vi "ADC_treat_data.vi"(1 "Inst_parameter":T1, 2 "data in":dbl[][](array[numeric])) -> (0 "data out":dbl[][](array[numeric]))   [LabVIEW 2013]
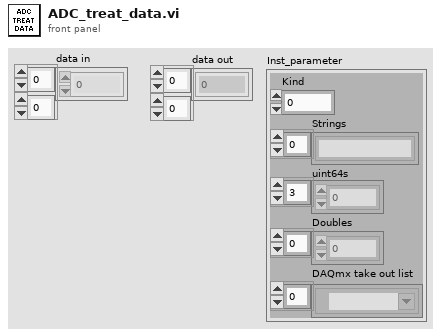
[diagram p1: front panel]
types:
  T1 = cluster{"Kind":u16, "Strings":string[], "uint64s":u64[], "Doubles":dbl[], "DAQmx take out list":refnum<k21>[]}
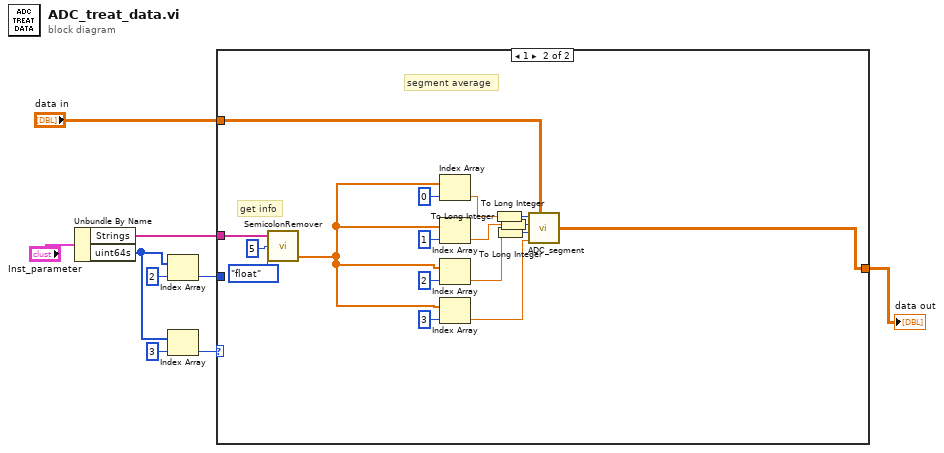
[diagram p0: block diagram]
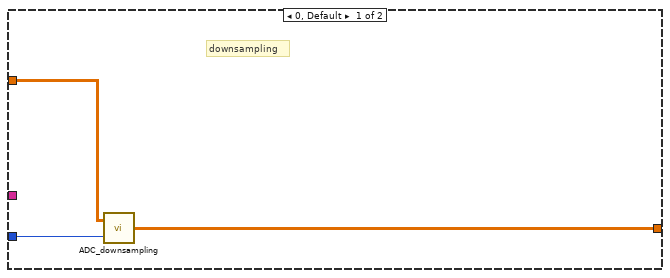
[diagram p2: hidden frame]
diagram:
  n1 = Unbundle By Name("Inst_parameter") -> ("Strings"=w6:string[], "uint64s"=w2:u64[])
  n2 = Index Array(array=w2, index=2) -> (element=w3:u64)
  n3 = Index Array(array=w2, index=3) -> (element=w5:u64)
  n4 = case shown="1" w5 {
    tunnel: "data in" -> [w11 w26]
    tunnel: w6 -> [_ w29]
    tunnel: w3 -> [w12 _]
    tunnel: [w10 w25] -> w1
    frame 0, Default {
      # "downsampling"
      n5 = call "ADC_downsampling.vi"("downsampling"=w12, "data in"=w11) -> ("data out"=w10:dbl[][])
    }
    frame 1 {
      # "get info"
      # "segment average"
      n6 = call "SemicolonRemover.vi"("output type"=enum16{"string", "int", "float"}."float", "index"=5, "Strings"=w29) -> ("float array"=w16:dbl[])  [unwired: 2 out]
      n7 = Index Array(array=w16, index=0) -> (element=w20:dbl)
      n8 = Index Array(array=w16, index=1) -> (element=w19:dbl)
      n9 = Index Array(array=w16, index=2) -> (element=w18:dbl)
      n10 = Index Array(array=w16, index=3) -> (element=w17:dbl)
      n11 = To Long Integer(number=w20) -> (32bit integer=w15:i32)
      n12 = To Long Integer(number=w18) -> (32bit integer=w13:i32)
      n13 = To Long Integer(number=w19) -> (32bit integer=w14:i32)
      n14 = call "ADC_segment.vi"("First point"=w15, "Segment Number"=w14, "Segment Length"=w13, "Segment Period"=w17, "data in"=w26) -> ("data out"=w25:dbl[][])
    }
  }
  "data out" <- w1
